vi "citas.vi"() -> ()   [LabVIEW 2016]
panel:
  out "Waveform Chart 6":dbl(graph)
  in  "Stop Button 6":bool
  out "Numeric Control 6":i32
  out "Waveform Chart 5":dbl(graph)
  in  "Stop Button 5":bool
  out "Numeric Control 5":i32
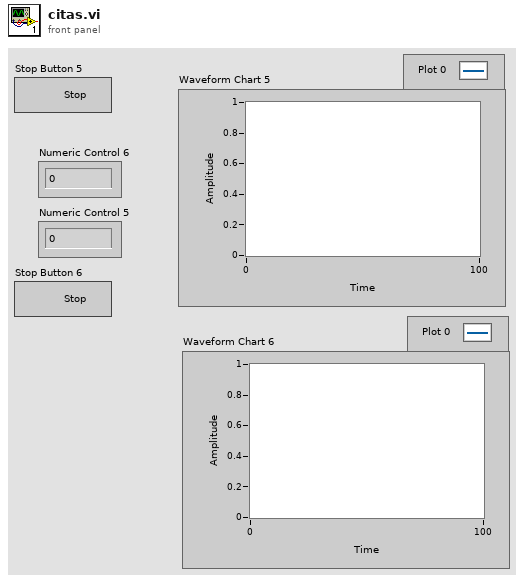
[diagram p1: front panel]
types:
  T1 = typedef "Rendezvous RefNum" = refnum<k1>
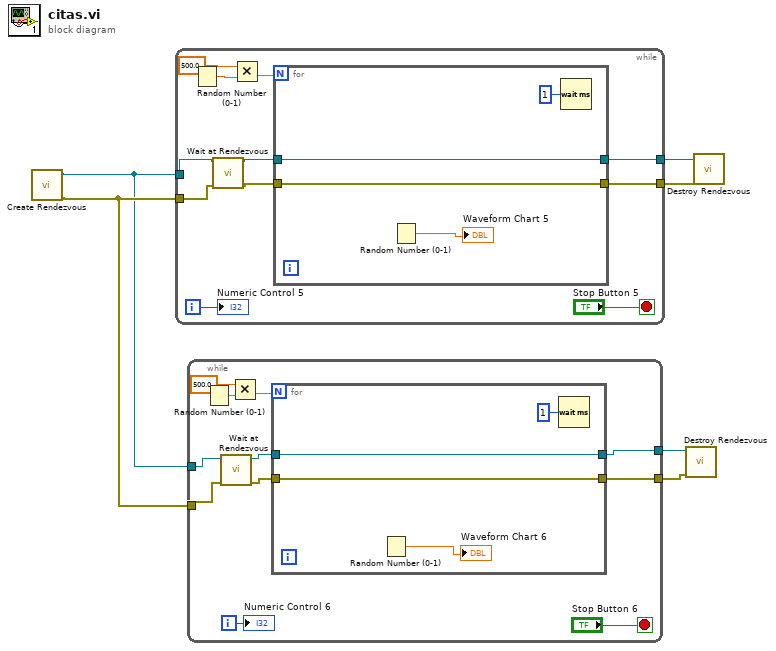
[diagram p0: block diagram]
diagram:
  n1 = call <vilib>:"Create Rendezvous.vi"() -> ("error out"=w6:errorcluster, "rendezvous"=w5:T1)  [unwired: 5 in, 1 out]
  n2 = while {
    tunnel: w5 -> [w12]
    tunnel: w6 -> [w11]
    tunnel: [w8] -> w4
    tunnel: [w7] -> w3
    i -> [w13]
    stop <- "Stop Button 5" stop-if-true
    n3 = Random Number (0-1)() -> (number: 0 to 1=w17:dbl)
    n4 = call <vilib>:"Wait at Rendezvous.vi"("error in (no error)"=w11, "rendezvous"=w12) -> ("error out"=w10:errorcluster, "rendezvous out"=w9:T1)  [unwired: 3 in, 1 out]
    n5 = Multiply(x=500.0, y=w17) -> (x*y=w15:dbl)
    n6 = for {
      N: w15 -> [_]
      tunnel: [w19] -> w8
      tunnel: w9 -> [w19]
      tunnel: [w18] -> w7
      tunnel: w10 -> [w18]
      n7 = Random Number (0-1)() -> (number: 0 to 1=→"Waveform Chart 5":dbl)
      n8 = Wait (ms)(milliseconds to wait=u32 1) -> ()  [unwired: 1 out]
    }
    "Numeric Control 5" <- w13
  }
  n9 = while {
    tunnel: w6 -> [w26]
    tunnel: w5 -> [w27]
    tunnel: [w23] -> w2
    tunnel: [w22] -> w1
    i -> [w28]
    stop <- "Stop Button 6" stop-if-true
    n10 = Random Number (0-1)() -> (number: 0 to 1=w32:dbl)
    n11 = call <vilib>:"Wait at Rendezvous.vi"("error in (no error)"=w26, "rendezvous"=w27) -> ("error out"=w24:errorcluster, "rendezvous out"=w25:T1)  [unwired: 3 in, 1 out]
    n12 = Multiply(x=500.0, y=w32) -> (x*y=w30:dbl)
    n13 = for {
      N: w30 -> [_]
      tunnel: [w34] -> w23
      tunnel: w25 -> [w34]
      tunnel: [w33] -> w22
      tunnel: w24 -> [w33]
      n14 = Random Number (0-1)() -> (number: 0 to 1=→"Waveform Chart 6":dbl)
      n15 = Wait (ms)(milliseconds to wait=u32 1) -> ()  [unwired: 1 out]
    }
    "Numeric Control 6" <- w28
  }
  n16 = call <vilib>:"Destroy Rendezvous.vi"("error in (no error)"=w1, "rendezvous"=w2) -> ()  [unwired: 4 in, 2 out]
  n17 = call <vilib>:"Destroy Rendezvous.vi"("error in (no error)"=w3, "rendezvous"=w4) -> ()  [unwired: 4 in, 2 out]
